vi "Untitled 2.vi"(0 "setpoint":dbl format="%.2f", 1 "output range":cluster{"output high":dbl, "output low":dbl}={"output high"=100.0, "output low"=-100.0} {"output low" format="%.2f"; "output high" format="%.2f"}, 5 "process variable":dbl format="%.2f", 7 "Initial integrated error":dbl, 9 "PID gains":T1={"proportional gain (Kc)"=1.0, "integral time (Ti, min)"=0.01, "derivative time (Td, min)"=0.0} {"derivative time (Td, min)" format="%.3f"; "integral time (Ti, min)" format="%.3f"; "proportional gain (Kc)" format="%.3f"}, 11 "dt (s)":dbl=-1.0 format="%.3f", 14 "reinitialize? (F)":bool) -> (4 "output":dbl format="%.2f", 15 "dt out (s)":dbl format="%.3f")   [LabVIEW 2016]
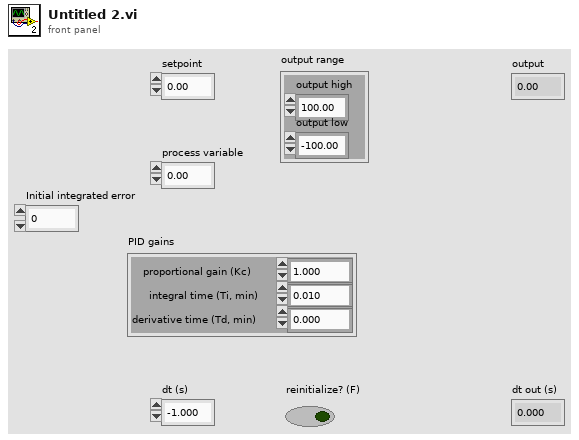
[diagram p1: front panel]
types:
  T1 = cluster{"proportional gain (Kc)":dbl, "integral time (Ti, min)":dbl, "derivative time (Td, min)":dbl}
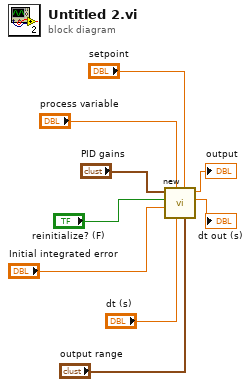
[diagram p0: block diagram]
diagram:
  n1 = call "new.vi"("output range"="output range", "setpoint"="setpoint", "dt (s)"="dt (s)", "process variable"="process variable", "Initial integrated error"="Initial integrated error", "reinitialize? (F)"="reinitialize? (F)", "PID gains"="PID gains") -> ("dt out (s)"=→"dt out (s)":dbl, "output"=→"output":dbl)  [unwired: 3 in]
